vi "Laser Fine Cutting.vi"(0 "configuration file path":path=path "C:/Users/admin/OneDrive/文档/Inlafa.CCV254.MES/System/All Config.ini" caption="配置文件的路径", 1 "fine cutting msic":T1) -> ()   [LabVIEW 2014]
uses:
  Ctl.xio/fine cutting msic ctl.ctl
  SubVIS.xio/DataSocket/DataSocket_Tags.ctl
  Ctl.xio/part type.ctl
  SubVIS.xio/DataSocket/Write PLC Vars/Write String Var in.vi
  <vilib>/Utility/file.llb/Read From Spreadsheet File (string).vi
  SubVIS.xio/DataSocket/Write PLC Vars/Write Bool Var in.vi
  SubVIS.xio/DataSocket/Read PLC Vars/Read String Var.vi
  SubVIS.xio/DataSocket/Write PLC Vars/Write Dbl Var in.vi
  SubVIS.xio/DataSocket/Read PLC Vars/Read Bool Var.vi
  SubVIS.xio/DataSocket/Read PLC Vars/Read U32 Var.vi
panel:
  in  "SQL information":string
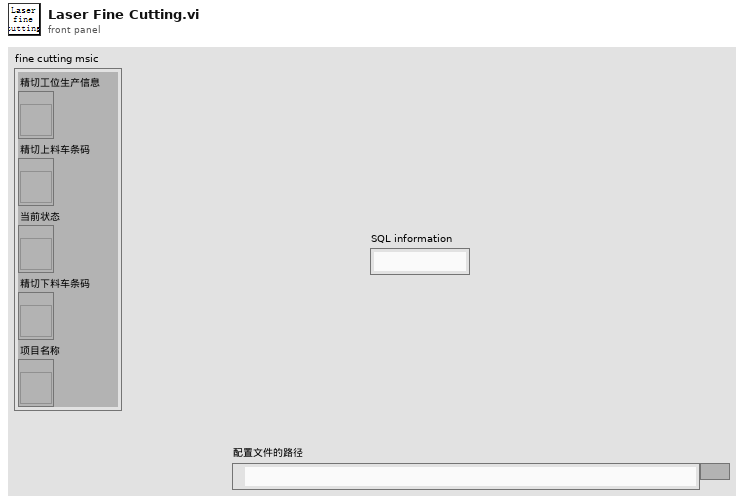
[diagram p1: front panel]
types:
  T1 = cluster{"精切工位生产信息":refnum<vi>, "精切上料车条码":refnum<vi>, "当前状态":refnum<vi>, "精切下料车条码":refnum<vi>, "项目名称":refnum<vi>}
  T2 = typedef "fine cutting msic ctl.ctl" = cluster{"configuration file path":path, "DsOut":T3[], "Hopper in car information":cluster{"Hopper car code":string, "Hopper car No":string, "plate No":string}, "pallet.produced number":i32, "SQL information":string, "Database":string[], "Serial number":i32, "database path":path, "fine cutting msic":cluster{"精切工位生产信息":refnum<vi>, "精切上料车条码":refnum<vi>, "当前状态":refnum<vi>, "精切下料车条码":refnum<vi>, "项目名称":refnum<vi>}, "part type":T4, "scanner1 coms or ip":string, "scanner2 coms or ip":string, "scanner1 resource name out":refnum<visa-resource-name>, "scanner2 resource name out":refnum<visa-resource-name>, "BarCode1":string, "BarCode2":string, "Hopper out information":cluster{"Hopper car code":string, "Hopper car No":string, "plate No":string}, "scanner1 ip ID":refnum<k5>, "scanner2 ip ID":refnum<k5>, "Number of scans":i32}
  T3 = typedef "DataSocket_Tags.ctl" = cluster{"Ds ID":refnum<k13>, "Tag":string}
  T4 = typedef "part type.ctl" = cluster{"项目号":string, "物料代码":string, "零件号":string, "供应商编码":string, "产线编码":string, "客户代码":string, "颜色代码":string, "托盘上限":i32, "加热温度":string, "加热时长":string, "EOL Stations":string}
  T5 = cluster{"Hopper car code":string, "Hopper car No":string, "plate No":string}
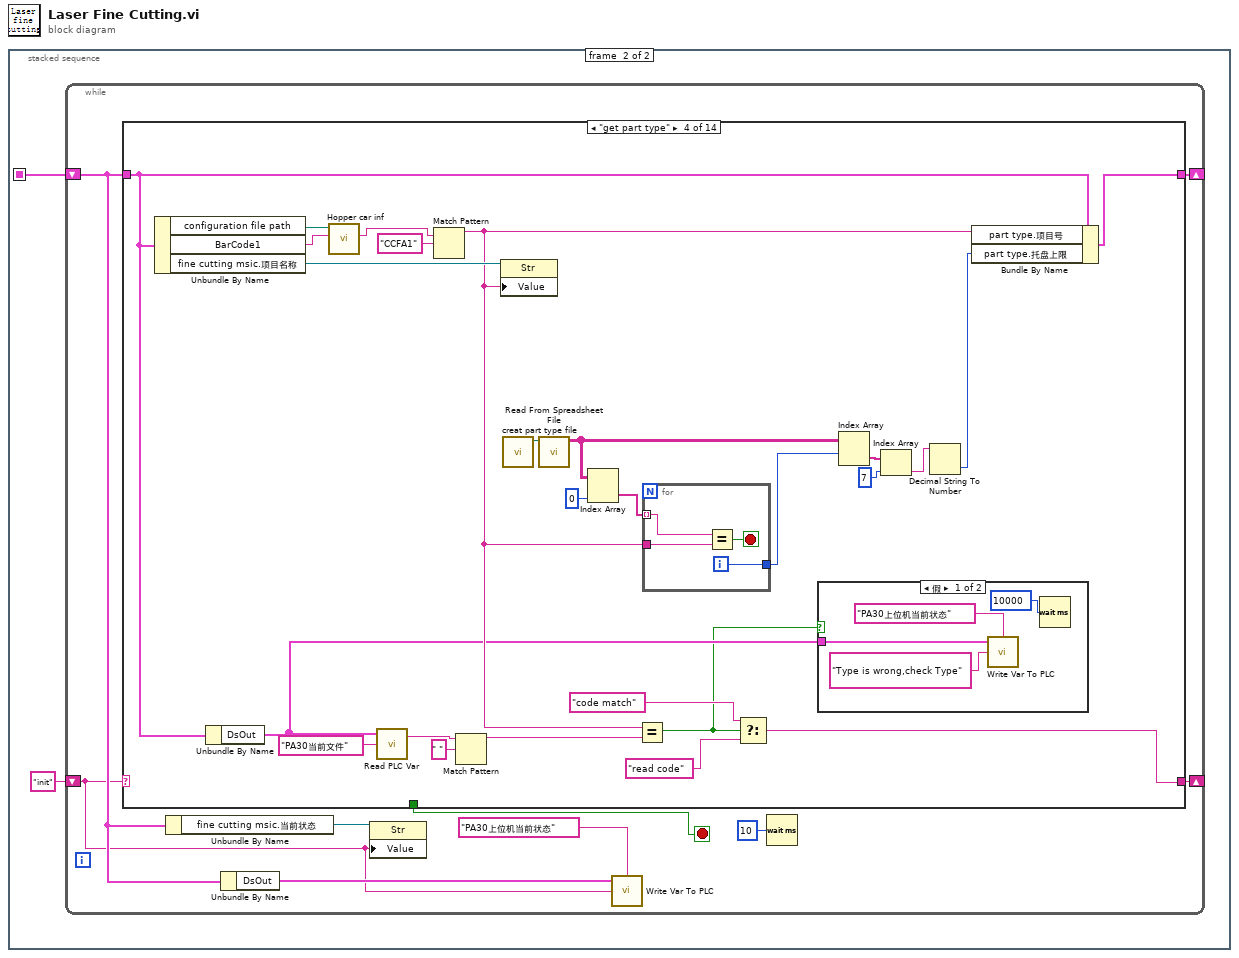
[diagram p0: block diagram]
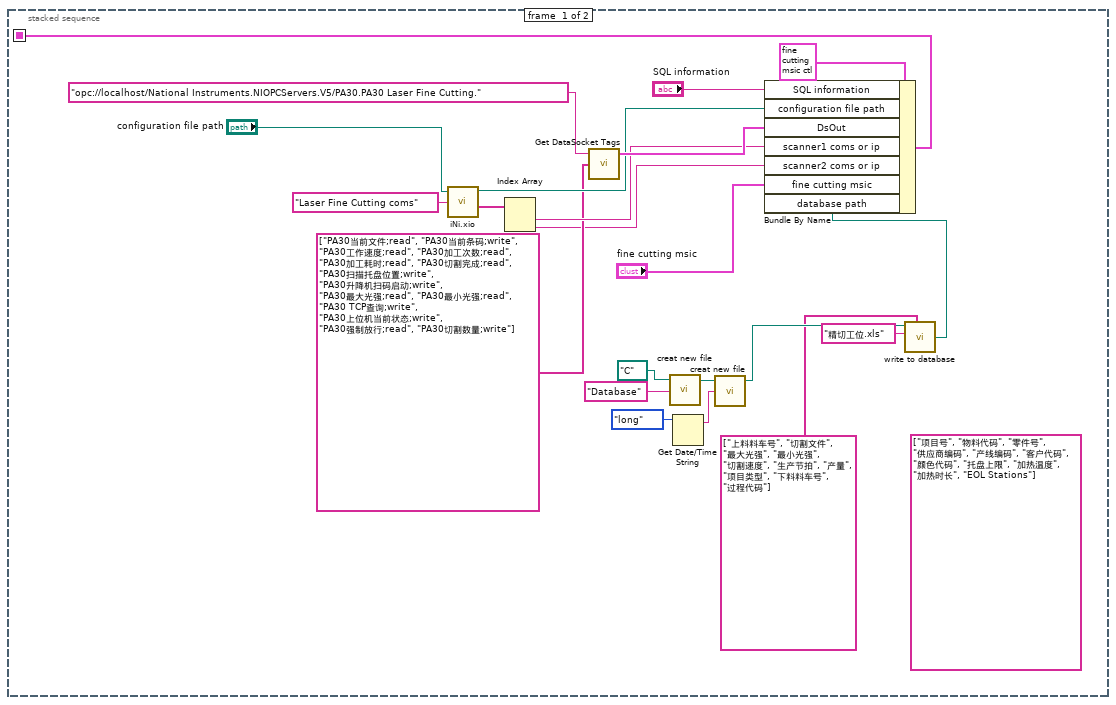
[diagram p2: hidden frame]
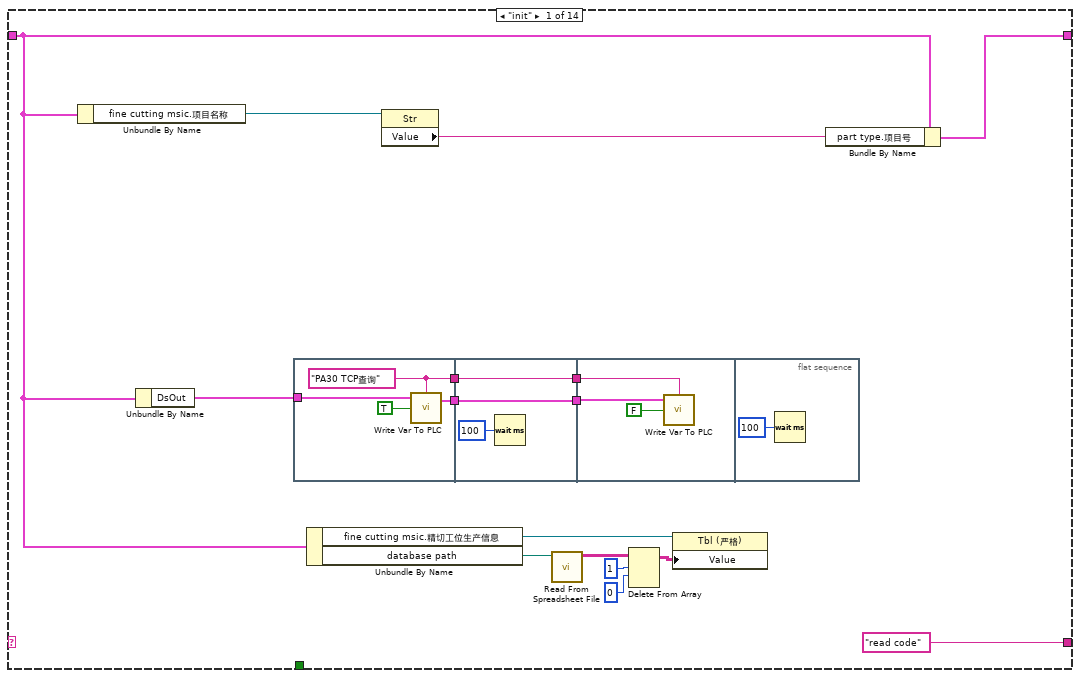
[diagram p3: hidden frame]
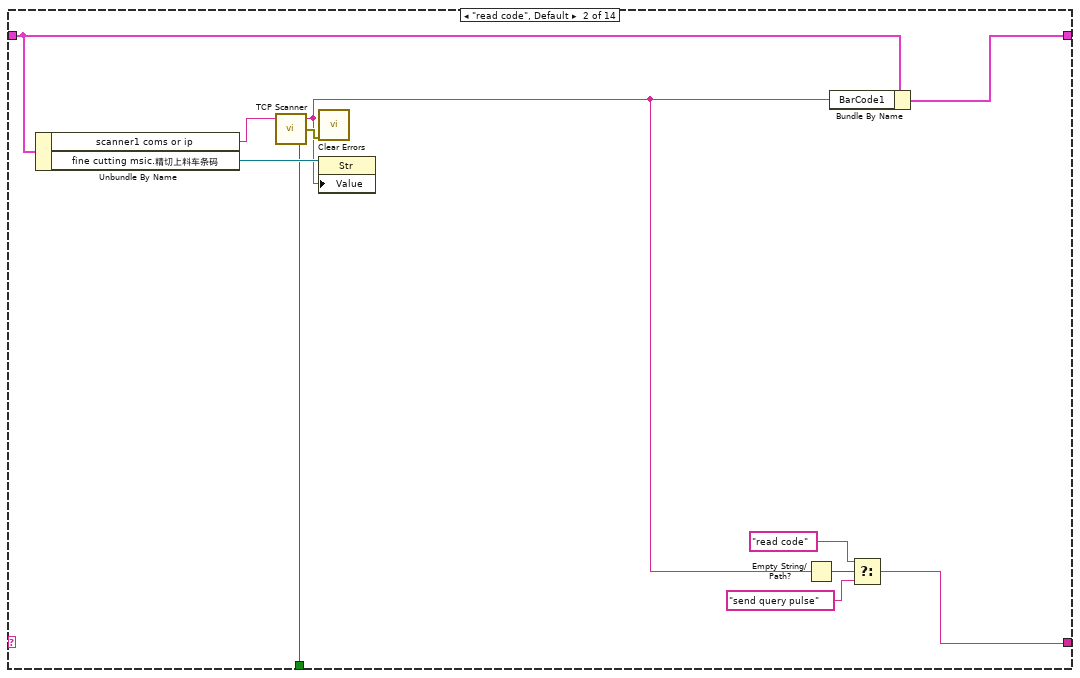
[diagram p4: hidden frame]
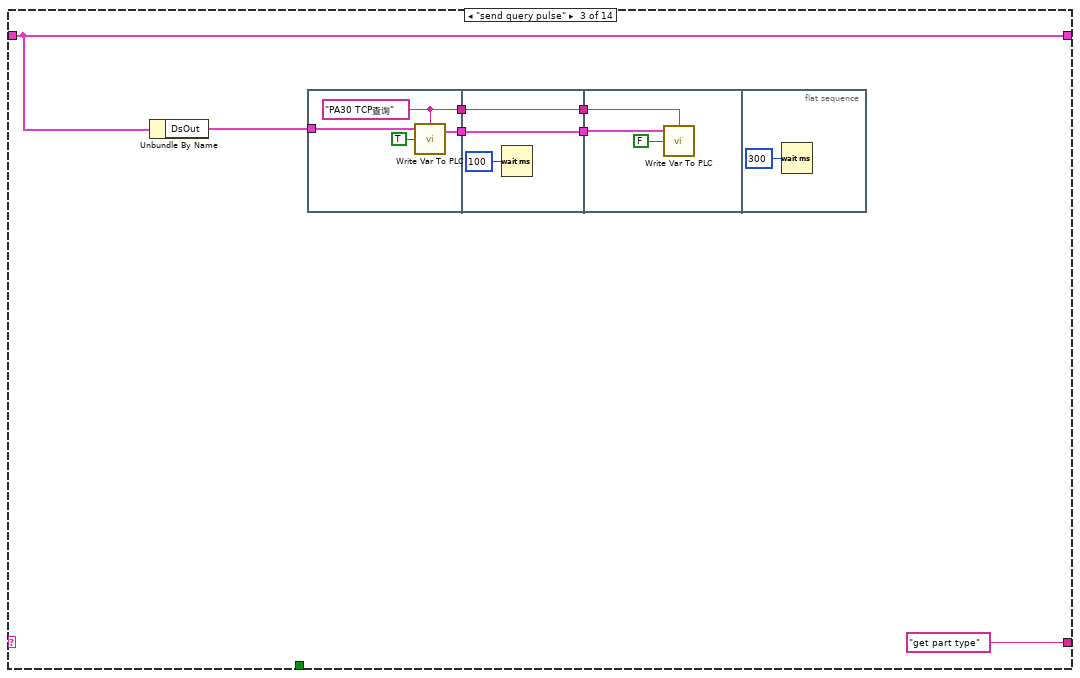
[diagram p5: hidden frame]
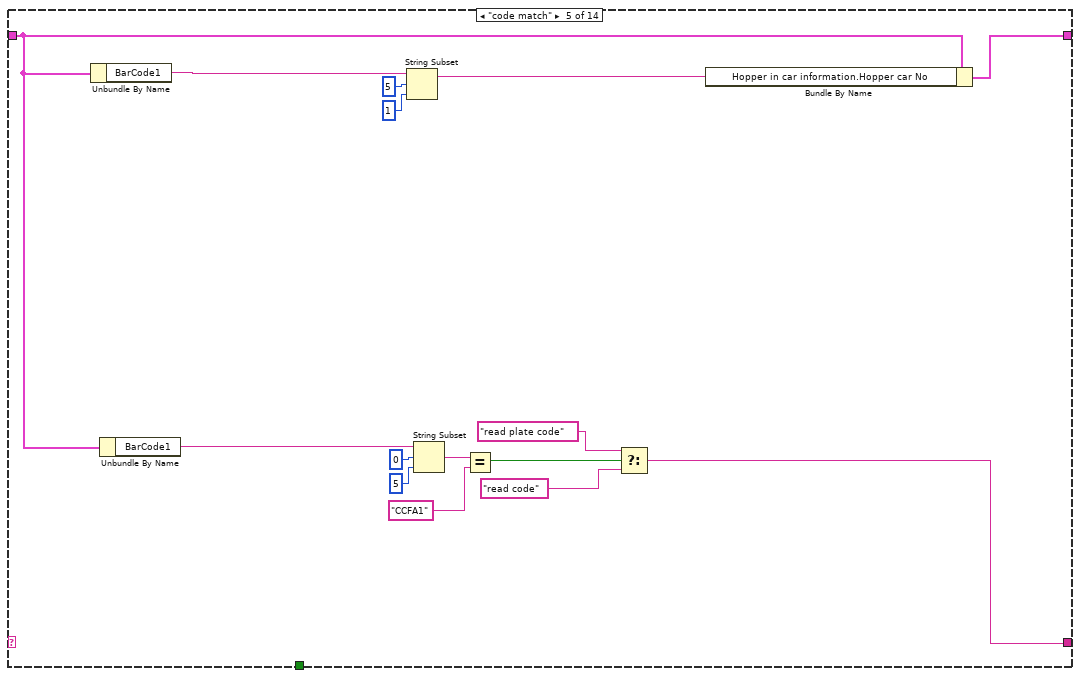
[diagram p7: hidden frame]
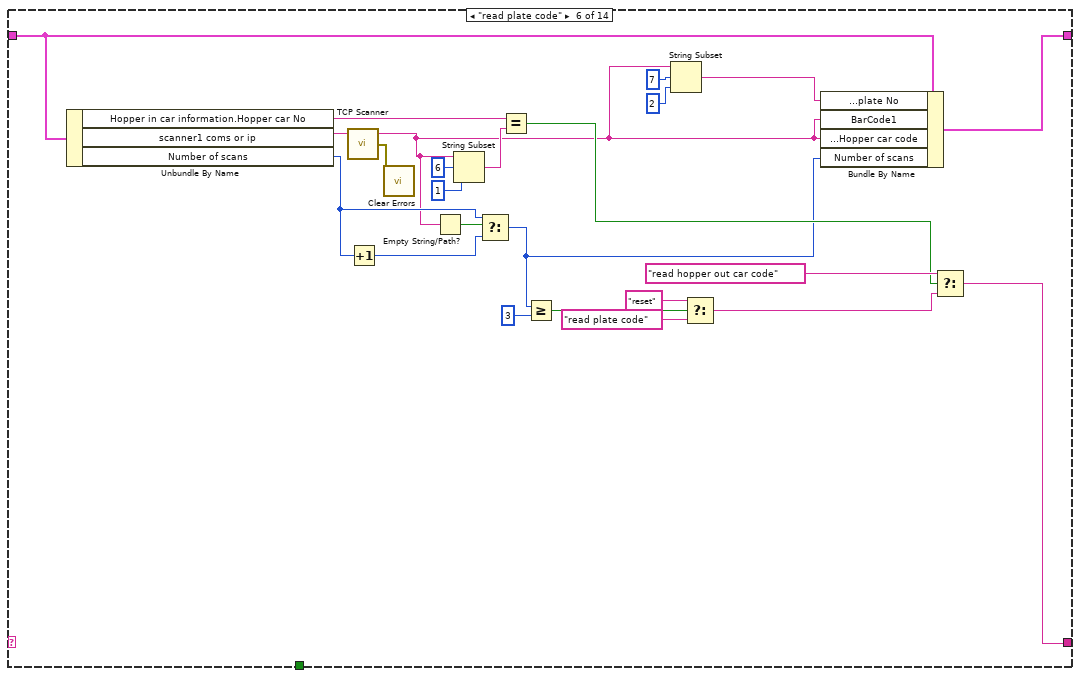
[diagram p8: hidden frame]
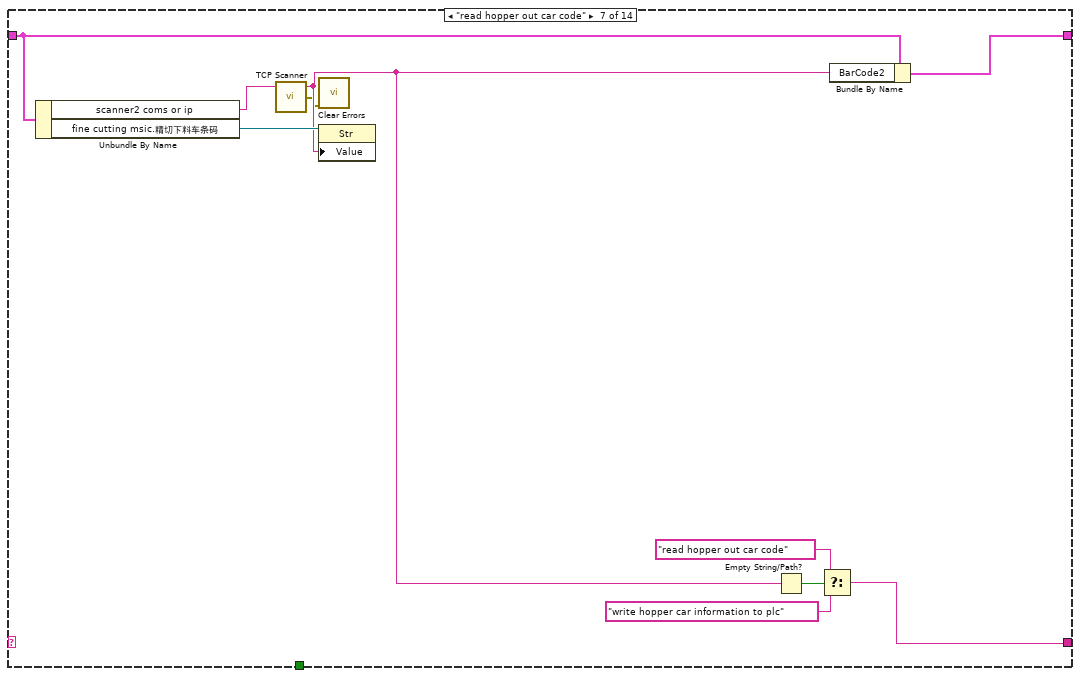
[diagram p9: hidden frame]
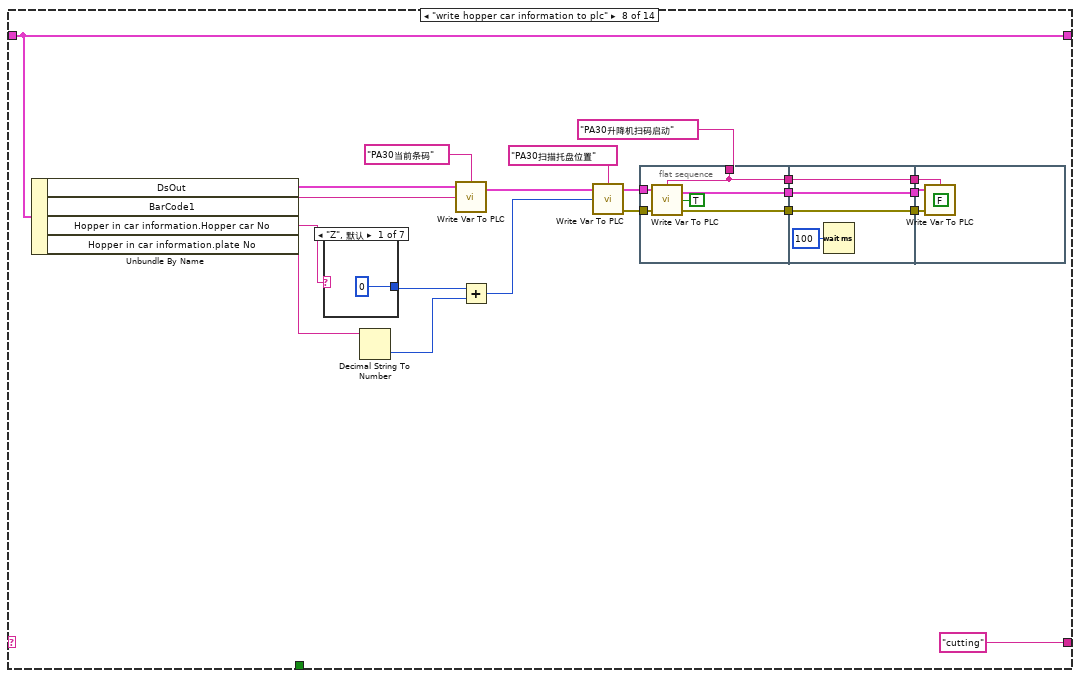
[diagram p10: hidden frame]
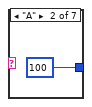
[diagram p11: hidden frame]
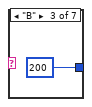
[diagram p12: hidden frame]
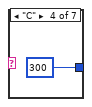
[diagram p13: hidden frame]
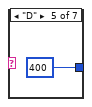
[diagram p14: hidden frame]
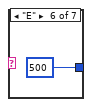
[diagram p15: hidden frame]
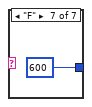
[diagram p16: hidden frame]
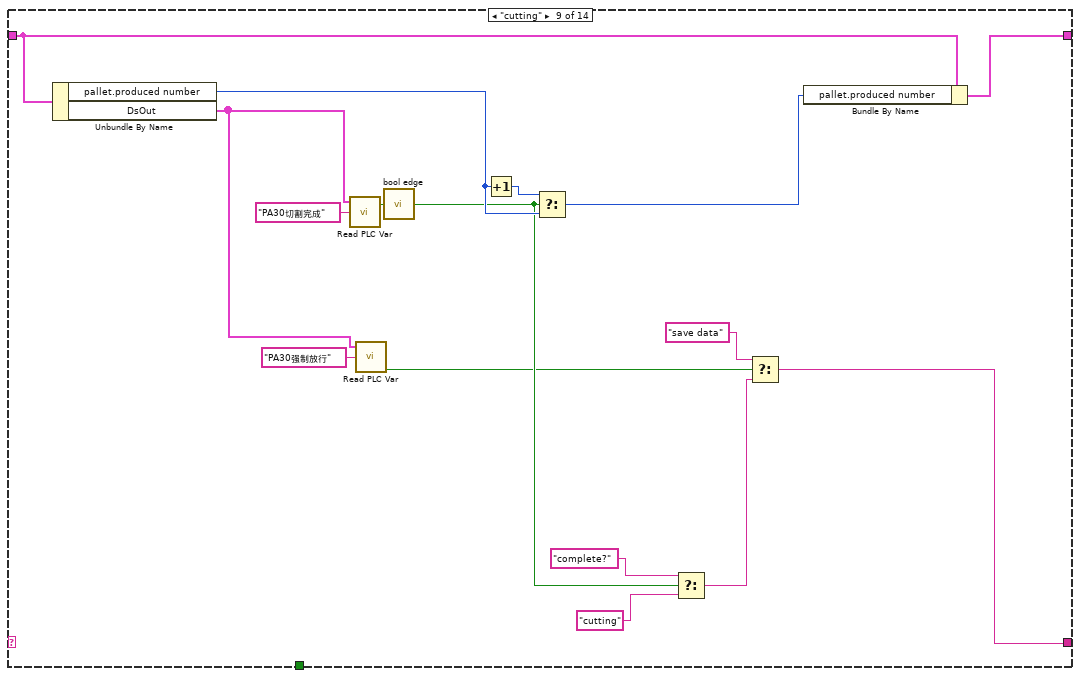
[diagram p17: hidden frame]
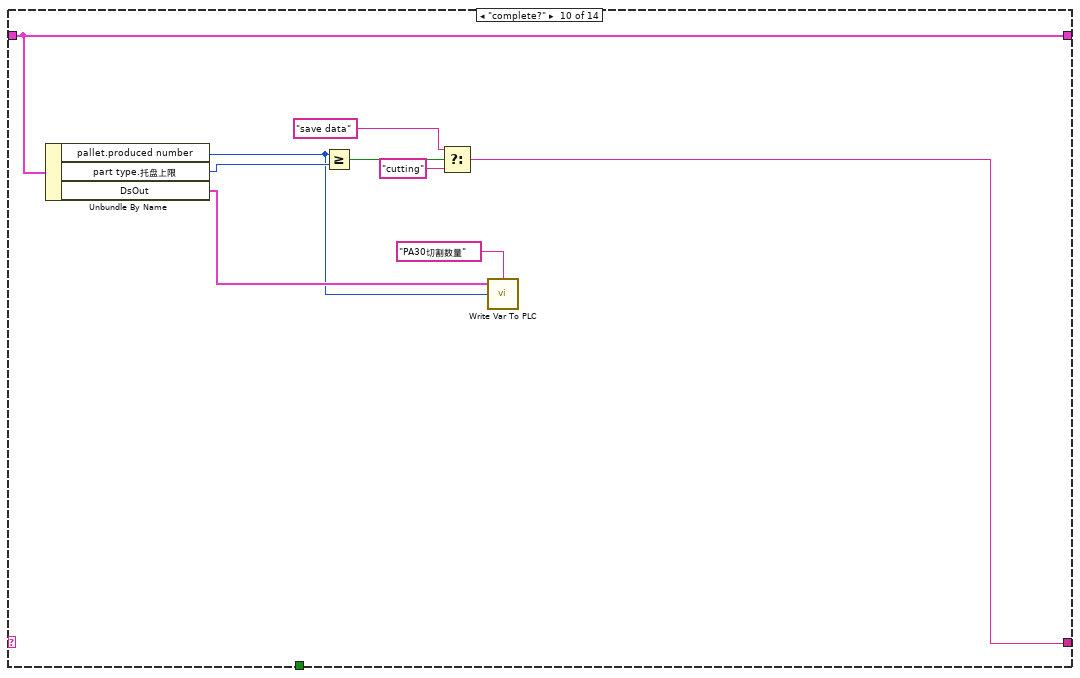
[diagram p18: hidden frame]
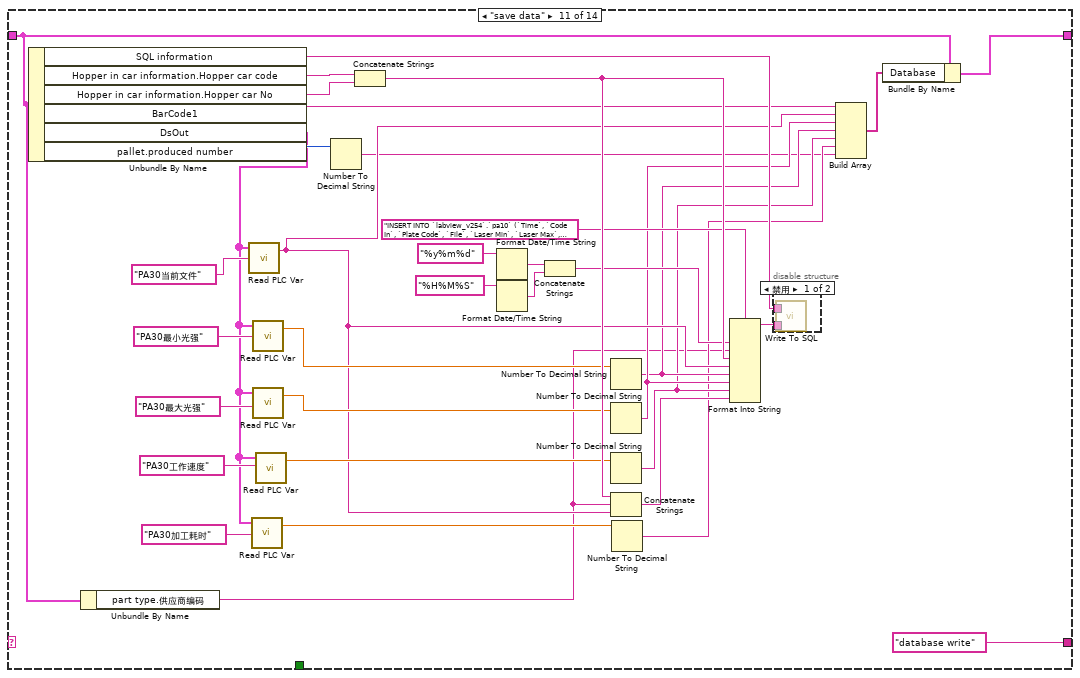
[diagram p19: hidden frame]
diagram:
  n1 = stacked-sequence {
    seq-local: [w10 _] -> [_ w23]
    frame #0 {
      (unwired) string[] ["项目号", "物料代码", "零件号", "供应商编码", "产线编码", "客户代码", "颜色代码", "托盘上限", "加热温度", "加热时长", "EOL Stations"]
      n2 = call "iNi.xio.vi"("configuration file path"="configuration file path", "Sections"="Laser Fine Cutting coms") -> ("configuration file path"=w21:path, "Values"=w19:string[])  [unwired: 1 in, 3 out]
      n3 = Index Array(array=w19) -> (element #1=w18:string, element #2=w12:string)  [unwired: 2 in]
      n4 = call "Get DataSocket Tags.vi"("All Tags"=string[] ["PA30当前文件;read", "PA30当前条码;write", "PA30工作速度;read", "PA30加工次数;read", "PA30加工耗时;read", "PA30切割完成;read", "PA30扫描托盘位置;write", "PA30升降机扫码启动;write", "PA30最大光强;read", "PA30最小光强;read", "PA30 TCP查询;write", "PA30上位机当前状态;write", "PA30强制放行;read", "PA30切割数量;write"], "URL"="opc://localhost/National Instruments.NIOPCServers.V5/PA30.PA30 Laser Fine Cutting.") -> ("DsOut"=w22:T3[])  [unwired: 3 in]
      n5 = call "creat new file.vi"("file name"="Database", "path"=path "C:/") -> ("created path"=w7:path)  [unwired: 1 in, 2 out]
      n6 = Get Date/Time String(date format (0)=enum16{"short", "long", "abbreviated"}."long" ("日期格式(0)")) -> (date string=w5:string)  [unwired: 2 in, 1 out]
      n7 = call "creat new file.vi"("file name"=w5, "path"=w7) -> ("created path"=w6:path)  [unwired: 1 in, 2 out]
      n8 = call "write to database.vi"("Header"=string[] ["上料料车号", "切割文件", "最大光强", "最小光强", "切割速度", "生产节拍", "产量", "项目类型", "下料料车号", "过程代码"], "file name"="精切工位.xls", "path"=w6) -> ("new file path (Not A Path if cancelled)"=w1:path)  [unwired: 3 in]
      n9 = Bundle By Name(cluster=T2 {"configuration file path"=path "", "DsOut"=[], "Hopper in car information"={"Hopper car code"="", "Hopper car No"="", "plate No"=""}, "pallet.produced number"=0, "SQL information"="", "Database"=[], "Serial number"=0, "database path"=path "", "fine cutting msic"={"精切工位生产信息"=refnum, "精切上料车条码"=refnum, "当前状态"=refnum, "精切下料车条码"=refnum, "项目名称"=refnum}, "part type"={"项目号"="", "物料代码"="", "零件号"="", "供应商编码"="", "产线编码"="", "客户代码"="", "颜色代码"="", "托盘上限"=0, "加热温度"="", "加热时长"="", "EOL Stations"=""}, "scanner1 coms or ip"="", "scanner2 coms or ip"="", "scanner1 resource name out"="", "scanner2 resource name out"="", "BarCode1"="", "BarCode2"="", "Hopper out information"={"Hopper car code"="", "Hopper car No"="", "plate No"=""}, "scanner1 ip ID"=refnum, "scanner2 ip ID"=refnum, "Number of scans"=0} ("rough cutting msic"), "SQL information"="SQL information", "configuration file path"=w21, "DsOut"=w22, "scanner1 coms or ip"=w18, "scanner2 coms or ip"=w12, "fine cutting msic"="fine cutting msic", "database path"=w1) -> (w10:T2)
    }
    frame #1 {
      n10 = while {
        shift-right: [w33] -> _
        shift-left: w23 -> [w28]
        shift-right: [w32] -> _
        shift-left: "init" ("event") -> [w26]
        stop <- w25 stop-if-true
        n11 = case shown="\"get part type\"" w26 {
          tunnel: w28 -> [w34 w69 w73 w97 w126 w151 w170 w173 w226 w234 w241 w295 w307 w315]
          tunnel: [w49 w71 w73 w115 w134 w148 w172 w173 w228 w234 w246 w296 w307 w320] -> w33
          tunnel: ["read code" w63 "get part type" ("f") w96 w132 w149 w165 "cutting" ("event") w215 w237 "database write" ("f") "updata display" ("f") "reset" ("f") "read code" ("f")] -> w32
          tunnel: [_ w61 _ _ _ _ _ _ _ _ _ _ _ _] -> w25
          frame "init" {
            n12 = Unbundle By Name(w34) -> ("fine cutting msic.项目名称"=w47:refnum<vi>)
            n13 = Unbundle By Name(w34) -> ("DsOut"=w41:T3[])
            n14 = flat-sequence {
              tunnel: w41 -> [w53]
              tunnel: [w51] -> w45
              tunnel: [w50] -> w44
              tunnel: w45 -> [w55]
              tunnel: [w55] -> w43
              tunnel: w44 -> [w54]
              tunnel: [w54] -> w42
              tunnel: w43 -> [w59]
              tunnel: w42 -> [w57]
              frame #0 {
                w50 = "PA30 TCP查询" ("Tag IN")
                n15 = call-poly "Write Var To PLC.vi"("Tag IN"=w50, "Bool Var in"=TRUE, "Ds PLCTags IN"=w53) -> ("Ds PLCTags OUT"=w51:T3[])  [unwired: 1 in, 1 out]
              }
              frame #1 {
                n16 = Wait (ms)(milliseconds to wait=u32 100 ("等待时间（毫秒）")) -> ()  [unwired: 1 out]
              }
              frame #2 {
                n17 = call-poly "Write Var To PLC.vi"("Tag IN"=w57, "Bool Var in"=FALSE, "Ds PLCTags IN"=w59) -> ()  [unwired: 1 in, 2 out]
              }
              frame #3 {
                n18 = Wait (ms)(milliseconds to wait=u32 100 ("等待时间（毫秒）")) -> ()  [unwired: 1 out]
              }
            }
            n19 = Unbundle By Name(w34) -> ("fine cutting msic.精切工位生产信息"=w40:refnum<vi>, "database path"=w39:path)
            n20 = property class="Str"(reference=w47) -> ("Value"=w46:string)  [unwired: 1 in, 2 out]
            n21 = call-poly <vilib>:"Read From Spreadsheet File.vi"("file path (dialog if empty)"=w39) -> ("all rows"=w38:string[][])  [unwired: 6 in, 4 out]
            n22 = Delete From Array(array=w38, length=1 ("长度"), index (row)=0 ("索引 (行)")) -> (array with subset deleted=w35:string[][])  [unwired: 1 in, 1 out]
            n23 = property class="Tbl (严格)"(reference=w40, "Value"=w35) -> ()  [unwired: 1 in, 2 out]
            n24 = Bundle By Name(cluster=w34, "part type.项目号"=w46) -> (w49:T2)
          }
          frame "read code", Default {
            n25 = Unbundle By Name(w69) -> ("scanner1 coms or ip"=w68:string, "fine cutting msic.精切上料车条码"=w70:refnum<vi>)
            n26 = call "TCP Scanner.vi"("ip"=w68) -> ("status"=w61:bool, "错误输出"=w67:errorcluster, "Barcode"=w62:string)  [unwired: 2 in]
            n27 = call <vilib>:"Clear Errors.vi"("error in (no error)"=w67) -> ()  [unwired: 5 in, 2 out]
            n28 = property class="Str"(reference=w70, "Value"=w62) -> ()  [unwired: 1 in, 2 out]
            n29 = Empty String/Path?(string/path=w62) -> (empty?=w66:bool)
            n30 = Bundle By Name(cluster=w69, "BarCode1"=w62) -> (w71:T2)
            n31 = Select(t="read code", s=w66, f="send query pulse") -> (s? t:f=w63:string)
          }
          frame "send query pulse" {
            n32 = Unbundle By Name(w73) -> ("DsOut"=w74:T3[])
            n33 = flat-sequence {
              tunnel: w74 -> [w82]
              tunnel: [w80] -> w78
              tunnel: [w79] -> w77
              tunnel: w78 -> [w84]
              tunnel: [w84] -> w76
              tunnel: w77 -> [w83]
              tunnel: [w83] -> w75
              tunnel: w76 -> [w88]
              tunnel: w75 -> [w86]
              frame #0 {
                w79 = "PA30 TCP查询" ("Tag IN")
                n34 = call-poly "Write Var To PLC.vi"("Tag IN"=w79, "Bool Var in"=TRUE, "Ds PLCTags IN"=w82) -> ("Ds PLCTags OUT"=w80:T3[])  [unwired: 1 in, 1 out]
              }
              frame #1 {
                n35 = Wait (ms)(milliseconds to wait=u32 100 ("等待时间（毫秒）")) -> ()  [unwired: 1 out]
              }
              frame #2 {
                n36 = call-poly "Write Var To PLC.vi"("Tag IN"=w86, "Bool Var in"=FALSE, "Ds PLCTags IN"=w88) -> ()  [unwired: 1 in, 2 out]
              }
              frame #3 {
                n37 = Wait (ms)(milliseconds to wait=u32 300 ("等待时间（毫秒）")) -> ()  [unwired: 1 out]
              }
            }
          }
          frame "get part type" {
            n38 = Unbundle By Name(w97) -> ("configuration file path"=w105:path, "BarCode1"=w104:string, "fine cutting msic.项目名称"=w103:refnum<vi>)
            n39 = Unbundle By Name(w97) -> ("DsOut"=w91:T3[])
            n40 = call "Hopper car inf.vi"("key"=w104, "path in"=w105) -> ("value out"=w102:string)  [unwired: 8 in, 1 out]
            n41 = call-poly "Read PLC Var.vi"("Tag IN"="PA30当前文件", "Ds PLCTags IN"=w91) -> ("String Var out"=w94:string)  [unwired: 1 in, 1 out]
            n42 = Match Pattern(string=w102, regular expression="CCFA1" ("正则表达式")) -> (before substring=w95:string)  [unwired: 1 in, 3 out]
            n43 = Match Pattern(string=w94, regular expression=" " ("正则表达式")) -> (before substring=w92:string)  [unwired: 1 in, 3 out]
            n44 = property class="Str"(reference=w103, "Value"=w95) -> ()  [unwired: 1 in, 2 out]
            n45 = call "creat part type file.vi"() -> ("new file path (Not A Path if cancelled)"=w106:path)  [unwired: 11 in]
            n46 = call-poly <vilib>:"Read From Spreadsheet File.vi"("file path (dialog if empty)"=w106) -> ("all rows"=w110:string[][])  [unwired: 6 in, 4 out]
            n47 = Index Array(array=w110, index (col)=0 ("禁用的索引 (列)")) -> (element=w111:string[])  [unwired: 1 in]
            n48 = Equal?(x=w95, y=w92) -> (x = y?=w90:bool)
            n49 = for {
              tunnel: w111 -> [w120] mode=indexing
              tunnel: [w122] -> w109
              tunnel: w95 -> [w121]
              i -> [w122]
              stop <- w123 stop-if-true
              n50 = Equal?(x=w120, y=w121) -> (x = y?=w123:bool)
            }
            n51 = Select(t="code match" ("event"), s=w90, f="read code" ("event")) -> (s? t:f=w96:string)
            n52 = case shown="假" w90 {
              tunnel: w91 -> [w119 _]
              frame False {
                n53 = call-poly "Write Var To PLC.vi"("Tag IN"="PA30上位机当前状态", "String Var in"="Type is wrong,check Type", "Ds PLCTags IN"=w119) -> ()  [unwired: 1 in, 2 out]
                n54 = Wait (ms)(milliseconds to wait=u32 10000 ("等待时间（毫秒）")) -> ()  [unwired: 1 out]
              }
              frame True {
              }
            }
            n55 = Index Array(array=w110, index (row)=w109) -> (element=w108:string[])  [unwired: 1 in]
            n56 = Index Array(array=w108, index=7 ("索引")) -> (element=w113:string)
            n57 = Decimal String To Number(string=w113) -> (number=w107:i32)  [unwired: 2 in, 1 out]
            n58 = Bundle By Name(cluster=w97, "part type.项目号"=w95, "part type.托盘上限"=w107) -> (w115:T2)
          }
          frame "code match" {
            n59 = Unbundle By Name(w126) -> ("BarCode1"=w127:string)
            n60 = Unbundle By Name(w126) -> ("BarCode1"=w125:string)
            n61 = String Subset(string=w127, offset (0)=5 ("偏移量(0)"), length (rest)=1 ("长度（剩余）")) -> (substring=w129:string)
            n62 = String Subset(string=w125, offset (0)=0 ("偏移量(0)"), length (rest)=5 ("长度（剩余）")) -> (substring=w130:string)
            n63 = Equal?(x=w130, y="CCFA1") -> (x = y?=w133:bool)
            n64 = Select(t="read plate code" ("event"), s=w133, f="read code" ("event")) -> (s? t:f=w132:string)
            n65 = Bundle By Name(cluster=w126, "Hopper in car information.Hopper car No"=w129) -> (w134:T2)
          }
          frame "read plate code" {
            n66 = Unbundle By Name(w151) -> ("Hopper in car information.Hopper car No"=w159:string, "scanner1 coms or ip"=w162:string, "Number of scans"=w145:i32)
            n67 = call "TCP Scanner.vi"("ip"=w162) -> ("错误输出"=w147:errorcluster, "Barcode"=w139:string)  [unwired: 2 in, 1 out]
            n68 = Increment(x=w145) -> (x+1=w144:i32)
            n69 = call <vilib>:"Clear Errors.vi"("error in (no error)"=w147) -> ()  [unwired: 5 in, 2 out]
            n70 = Empty String/Path?(string/path=w139) -> (empty?=w146:bool)
            n71 = String Subset(string=w139, offset (0)=6 ("偏移量(0)"), length (rest)=1 ("长度（剩余）")) -> (substring=w156:string)
            n72 = Select(t=w145, s=w146, f=w144) -> (s? t:f=w143:i32)
            n73 = Equal?(x=w159, y=w156) -> (x = y?=w157:bool)
            n74 = Greater Or Equal?(x=w143, y=3) -> (x >= y?=w155:bool)
            n75 = String Subset(string=w139, offset (0)=7 ("偏移量(0)"), length (rest)=2 ("长度（剩余）")) -> (substring=w140:string)
            n76 = Select(t="reset" ("event"), s=w155, f="read plate code" ("event")) -> (s? t:f=w152:string)
            n77 = Bundle By Name(cluster=w151, "Hopper in car information.plate No"=w140, "BarCode1"=w139, "Hopper in car information.Hopper car code"=w139, "Number of scans"=w143) -> (w148:T2)
            n78 = Select(t="read hopper out car code" ("event"), s=w157, f=w152) -> (s? t:f=w149:string)
          }
          frame "read hopper out car code" {
            n79 = Unbundle By Name(w170) -> ("scanner2 coms or ip"=w164:string, "fine cutting msic.精切下料车条码"=w171:refnum<vi>)
            n80 = call "TCP Scanner.vi"("ip"=w164) -> ("错误输出"=w163:errorcluster, "Barcode"=w169:string)  [unwired: 2 in, 1 out]
            n81 = call <vilib>:"Clear Errors.vi"("error in (no error)"=w163) -> ()  [unwired: 5 in, 2 out]
            n82 = property class="Str"(reference=w171, "Value"=w169) -> ()  [unwired: 1 in, 2 out]
            n83 = Empty String/Path?(string/path=w169) -> (empty?=w168:bool)
            n84 = Select(t="read hopper out car code" ("f"), s=w168, f="write hopper car information to plc") -> (s? t:f=w165:string)
            n85 = Bundle By Name(cluster=w170, "BarCode2"=w169) -> (w172:T2)
          }
          frame "write hopper car information to plc" {
            n86 = Unbundle By Name(w173) -> ("DsOut"=w176:T3[], "BarCode1"=w175:string, "Hopper in car information.Hopper car No"=w193:string, "Hopper in car information.plate No"=w192:string)
            n87 = case shown="\"Z\", 默认" w193 {
              tunnel: [0 100 200 300 400 500 600] -> w191
              frame "Z", Default {
              }
              frame "A" {
              }
              frame "B" {
              }
              frame "C" {
              }
              frame "D" {
              }
              frame "E" {
              }
              frame "F" {
              }
            }
            n88 = Decimal String To Number(string=w192) -> (number=w190:i32)  [unwired: 2 in, 1 out]
            n89 = call-poly "Write Var To PLC.vi"("Tag IN"="PA30当前条码", "String Var in"=w175, "Ds PLCTags IN"=w176) -> ("Ds PLCTags OUT"=w177:T3[])  [unwired: 1 in, 1 out]
            n90 = Add(x=w191, y=w190) -> (x+y=w188:i32)
            n91 = call-poly "Write Var To PLC.vi"("Tag IN"="PA30扫描托盘位置", "Dbl Var in"=w188, "Ds PLCTags IN"=w177) -> ("error out"=w187:errorcluster, "Ds PLCTags OUT"=w186:T3[])  [unwired: 1 in]
            n92 = flat-sequence {
              tunnel: w187 -> [w199]
              tunnel: w186 -> [w198]
              tunnel: "PA30升降机扫码启动" ("Tag IN") -> [w195]
              tunnel: [w196] -> w182
              tunnel: [w195] -> w181
              tunnel: [w194] -> w179
              tunnel: [w202] -> w183
              tunnel: w182 -> [w202]
              tunnel: w181 -> [w201]
              tunnel: [w201] -> w180
              tunnel: w179 -> [w200]
              tunnel: [w200] -> w178
              tunnel: w183 -> [w207]
              tunnel: w180 -> [w206]
              tunnel: w178 -> [w205]
              frame #0 {
                n93 = call-poly "Write Var To PLC.vi"("Tag IN"=w195, "错误输入（无错误）"=w199, "Bool Var in"=TRUE, "Ds PLCTags IN"=w198) -> ("error out"=w194:errorcluster, "Ds PLCTags OUT"=w196:T3[])
              }
              frame #1 {
                n94 = Wait (ms)(milliseconds to wait=u32 100 ("等待时间（毫秒）")) -> ()  [unwired: 1 out]
              }
              frame #2 {
                n95 = call-poly "Write Var To PLC.vi"("Tag IN"=w206, "错误输入（无错误）"=w205, "Bool Var in"=FALSE, "Ds PLCTags IN"=w207) -> ()  [unwired: 2 out]
              }
            }
          }
          frame "cutting" {
            n96 = Unbundle By Name(w226) -> ("pallet.produced number"=w229:i32, "DsOut"=w219:T3[])
            n97 = call-poly "Read PLC Var.vi"("Tag IN"="PA30切割完成", "Ds PLCTags IN"=w219) -> ("Bool Var out"=w221:bool)  [unwired: 1 in, 1 out]
            n98 = call-poly "Read PLC Var.vi"("Tag IN"="PA30强制放行", "Ds PLCTags IN"=w219) -> ("Bool Var out"=w218:bool)  [unwired: 1 in, 1 out]
            n99 = call "bool edge.vi"("bool in"=w221) -> ("true-false"=w225:bool)  [unwired: 6 in, 1 out]
            n100 = Increment(x=w229) -> (x+1=w230:i32)
            n101 = Select(t=w230, s=w225, f=w229) -> (s? t:f=w227:i32)
            n102 = Select(t="complete?" ("event"), s=w225, f="cutting" ("event")) -> (s? t:f=w216:string)
            n103 = Select(t="save data" ("event"), s=w218, f=w216) -> (s? t:f=w215:string)
            n104 = Bundle By Name(cluster=w226, "pallet.produced number"=w227) -> (w228:T2)
          }
          frame "complete?" {
            n105 = Unbundle By Name(w234) -> ("pallet.produced number"=w231:i32, "part type.托盘上限"=w239:i32, "DsOut"=w232:T3[])
            n106 = Greater Or Equal?(x=w231, y=w239) -> (x >= y?=w238:bool)
            n107 = Select(t="save data" ("event"), s=w238, f="cutting") -> (s? t:f=w237:string)
            n108 = call-poly "Write Var To PLC.vi"("Tag IN"="PA30切割数量", "Dbl Var in"=w231, "Ds PLCTags IN"=w232) -> ()  [unwired: 1 in, 2 out]
          }
          frame "save data" {
            n109 = Unbundle By Name(w241) -> ("SQL information"=w256:string, "Hopper in car information.Hopper car code"=w258:string, "Hopper in car information.Hopper car No"=w257:string, "BarCode1"=w243:string, "DsOut"=w242:T3[], "pallet.produced number"=w245:i32)
            n110 = Unbundle By Name(w241) -> ("part type.供应商编码"=w240:string)
            n111 = call-poly "Read PLC Var.vi"("Tag IN"="PA30当前文件", "Ds PLCTags IN"=w242) -> ("String Var out"=w254:string)  [unwired: 1 in, 1 out]
            n112 = call-poly "Read PLC Var.vi"("Tag IN"="PA30加工耗时", "Ds PLCTags IN"=w242) -> ("U32 Var out"=w249:dbl)  [unwired: 1 in, 1 out]
            n113 = call-poly "Read PLC Var.vi"("Tag IN"="PA30最小光强", "Ds PLCTags IN"=w242) -> ("U32 Var out"=w263:dbl)  [unwired: 1 in, 1 out]
            n114 = call-poly "Read PLC Var.vi"("Tag IN"="PA30最大光强", "Ds PLCTags IN"=w242) -> ("U32 Var out"=w261:dbl)  [unwired: 1 in, 1 out]
            n115 = call-poly "Read PLC Var.vi"("Tag IN"="PA30工作速度", "Ds PLCTags IN"=w242) -> ("U32 Var out"=w259:dbl)  [unwired: 1 in, 1 out]
            n116 = Number To Decimal String(number=w245) -> (decimal integer string=w244:string)  [unwired: 1 in]
            n117 = Concatenate Strings(w258, w257) -> (w274:string)
            n118 = Format Date/Time String(time format string (%c)="%y%m%d" ("时间格式字符串(%c)")) -> (date/time string=w269:string)  [unwired: 2 in]
            n119 = Format Date/Time String(time format string (%c)="%H%M%S" ("时间格式字符串(%c)")) -> (date/time string=w268:string)  [unwired: 2 in]
            n120 = Concatenate Strings(w269, w268) -> (w266:string)
            n121 = Number To Decimal String(number=w263) -> (decimal integer string=w252:string)  [unwired: 1 in]
            n122 = Number To Decimal String(number=w261) -> (decimal integer string=w253:string)  [unwired: 1 in]
            n123 = Number To Decimal String(number=w259) -> (decimal integer string=w251:string)  [unwired: 1 in]
            n124 = Concatenate Strings(w274, w240, w254) -> (w271:string)
            n125 = Number To Decimal String(number=w249) -> (decimal integer string=w248:string)  [unwired: 1 in]
            n126 = Format Into String(format string="INSERT INTO `labview_v254`.`pa10` (`Time`, `Code In`, `Plate Code`, `File`, `Laser Min`, `Laser Max`, `Vel`, `Code Out`) VALUES ('%s', '%s', '%s', '%s', '%s', '%s', '%s', '%s');", w266, w240, w274, w254, w252, w253, w251, w271) -> (resulting string=w272:string)  [unwired: 2 in, 1 out]
            n127 = disable-structure shown="禁用" {
              disable-tunnel: w272 -> [w276 _]
              disable-tunnel: w256 -> [w275 _]
              frame Disabled {
                n128 = call "Write To SQL.vi"("SQL query"=w276, "connection information"=w275) -> ()  [unwired: 1 out]
              }
              frame Enabled {
              }
            }
            n129 = Build Array(w243, w254, w253, w252, w251, w248, w244) -> (w247:string[])
            n130 = Bundle By Name(cluster=w241, "Database"=w247) -> (w246:T2)
          }
          frame "database write" {
            n131 = Unbundle By Name(w295) -> ("Database"=w290:string[], "part type.项目号"=w289:string, "configuration file path"=w287:path, "Hopper in car information.Hopper car code"=w286:string, "BarCode2"=w285:string)
            n132 = Format Date/Time String(time format string (%c)="%y%m%d" ("时间格式字符串(%c)")) -> (date/time string=w281:string)  [unwired: 2 in]
            n133 = Format Date/Time String(time format string (%c)="%H%M%S" ("时间格式字符串(%c)")) -> (date/time string=w280:string)  [unwired: 2 in]
            n134 = call "Hopper car inf.vi"("key"=w286, "path in"=w287) -> ("value out"=w284:string, "path out"=w283:path)  [unwired: 8 in]
            n135 = Concatenate Strings(w281, w280) -> (w278:string)
            n136 = call "Hopper car inf.vi"("write\\read（read)"=enum16{"read", "write"}."write" ("write\\read（read)"), "value"=w284, "key"=w285, "path in"=w283) -> ()  [unwired: 6 in, 2 out]
            n137 = call "creat new file.vi"("file name"="Database", "path"=path "C:/") -> ("created path"=w294:path)  [unwired: 1 in, 2 out]
            n138 = Get Date/Time String(date format (0)=enum16{"short", "long", "abbreviated"}."long" ("日期格式(0)")) -> (date string=w292:string)  [unwired: 2 in, 1 out]
            n139 = Build Array (concatenate)(w290, w289, w285, w284, w278) -> (w288:string[])
            n140 = call "creat new file.vi"("file name"=w292, "path"=w294) -> ("created path"=w293:path)  [unwired: 1 in, 2 out]
            n141 = call "write to database.vi"("Header"=string[] ["上料料车号", "切割文件", "最大光强", "最小光强", "切割速度", "生产节拍", "产量", "项目类型", "下料料车号", "过程代码", "切割时间"], "data in"=w288, "file name"="精切工位.xls", "path"=w293) -> ("new file path (Not A Path if cancelled)"=w297:path)  [unwired: 2 in]
            n142 = Bundle By Name(cluster=w295, "database path"=w297) -> (w296:T2)
          }
          frame "updata display" {
            n143 = Unbundle By Name(w307) -> ("fine cutting msic.精切工位生产信息"=w309:refnum<vi>, "database path"=w308:path)
            n144 = call-poly <vilib>:"Read From Spreadsheet File.vi"("file path (dialog if empty)"=w308) -> ("all rows"=w306:string[][])  [unwired: 6 in, 4 out]
            n145 = Delete From Array(array=w306, length=1 ("长度"), index (row)=0 ("索引 (行)")) -> (array with subset deleted=w303:string[][])  [unwired: 1 in, 1 out]
            n146 = property class="Tbl (严格)"(reference=w309, "Value"=w303) -> ()  [unwired: 1 in, 2 out]
          }
          frame "reset" {
            w312 = ""
            w316 = "" ("BarCode")
            n147 = Unbundle By Name(w315) -> ("fine cutting msic.精切上料车条码"=w314:refnum<vi>, "fine cutting msic.精切下料车条码"=w313:refnum<vi>)
            n148 = property class="Str"(reference=w314, "Value"=w312) -> ()  [unwired: 1 in, 2 out]
            n149 = property class="Str"(reference=w313, "Value"=w312) -> ()  [unwired: 1 in, 2 out]
            n150 = Bundle By Name(cluster=w315, "Number of scans"=0, "pallet.produced number"=0, "BarCode1"=w316, "BarCode2"=w316, "Database"=string[] [], "Hopper in car information"=T5 {"Hopper car code"="", "Hopper car No"="", "plate No"=""} ("Hopper car information")) -> (w320:T2)
          }
        }
        n151 = Unbundle By Name(w28) -> ("fine cutting msic.当前状态"=w30:refnum<vi>)
        n152 = Unbundle By Name(w28) -> ("DsOut"=w27:T3[])
        n153 = property class="Str"(reference=w30, "Value"=w26) -> ()  [unwired: 1 in, 2 out]
        n154 = call-poly "Write Var To PLC.vi"("Tag IN"="PA30上位机当前状态", "String Var in"=w26, "Ds PLCTags IN"=w27) -> ()  [unwired: 1 in, 2 out]
        n155 = Wait (ms)(milliseconds to wait=u32 10 ("等待时间（毫秒）")) -> ()  [unwired: 1 out]
      }
    }
  }
